vi "Volt Freq Tach Properties.vi"(8 "error in":errorcluster, 10 "MeasType":T1, 11 "Rings Supported In":variant) -> (0 "error out":errorcluster, 3 "Rings Supported Out":variant)   [LabVIEW 2012]
uses:
  Custom Ctrls/ge_MeasType.ctl
  Custom Ctrls/ge_RingSupport.ctl
  Controls/HeaderNames.ctl
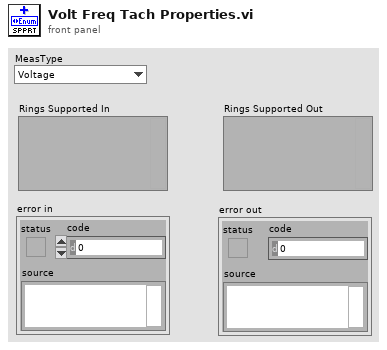
[diagram p1: front panel]
types:
  T1 = typedef "ge_MeasType.ctl" = enum16{"Voltage", "Frequency", "Tachometer", "Dynamic", "Thermocouple", "RTD", "Strain", "Current", "Resistance"}
  T2 = typedef "HeaderNames.ctl" = enum16{"Channel", "Device", "Spacer", "Description", "MB", "Range", "Terminal", "Coupling", "Thresh (V)", "Pulse/Rev", "Slope", "Min EU", "Min RPM", "mV/EU", "Iex", "Temp Units", "Type", "CJC Src", "CJC Val", "Ro", "Wire Cfg", "Strain Mode", "Vex", "Bridge Type", "GF", "Gauge Res", "Poisson", "Lead Res", "Init Strain", "GAF", "Scale", "Offset", "Unit (EU)", "dB?", "dB Ref", "Cal Mag", "Cal Units", "Max Temp", "Min Temp", "Max Strain", "Min Strain"}
  T3 = typedef "ge_RingSupport.ctl" = cluster{"Hdr Name":T2, "Values":u16[]}
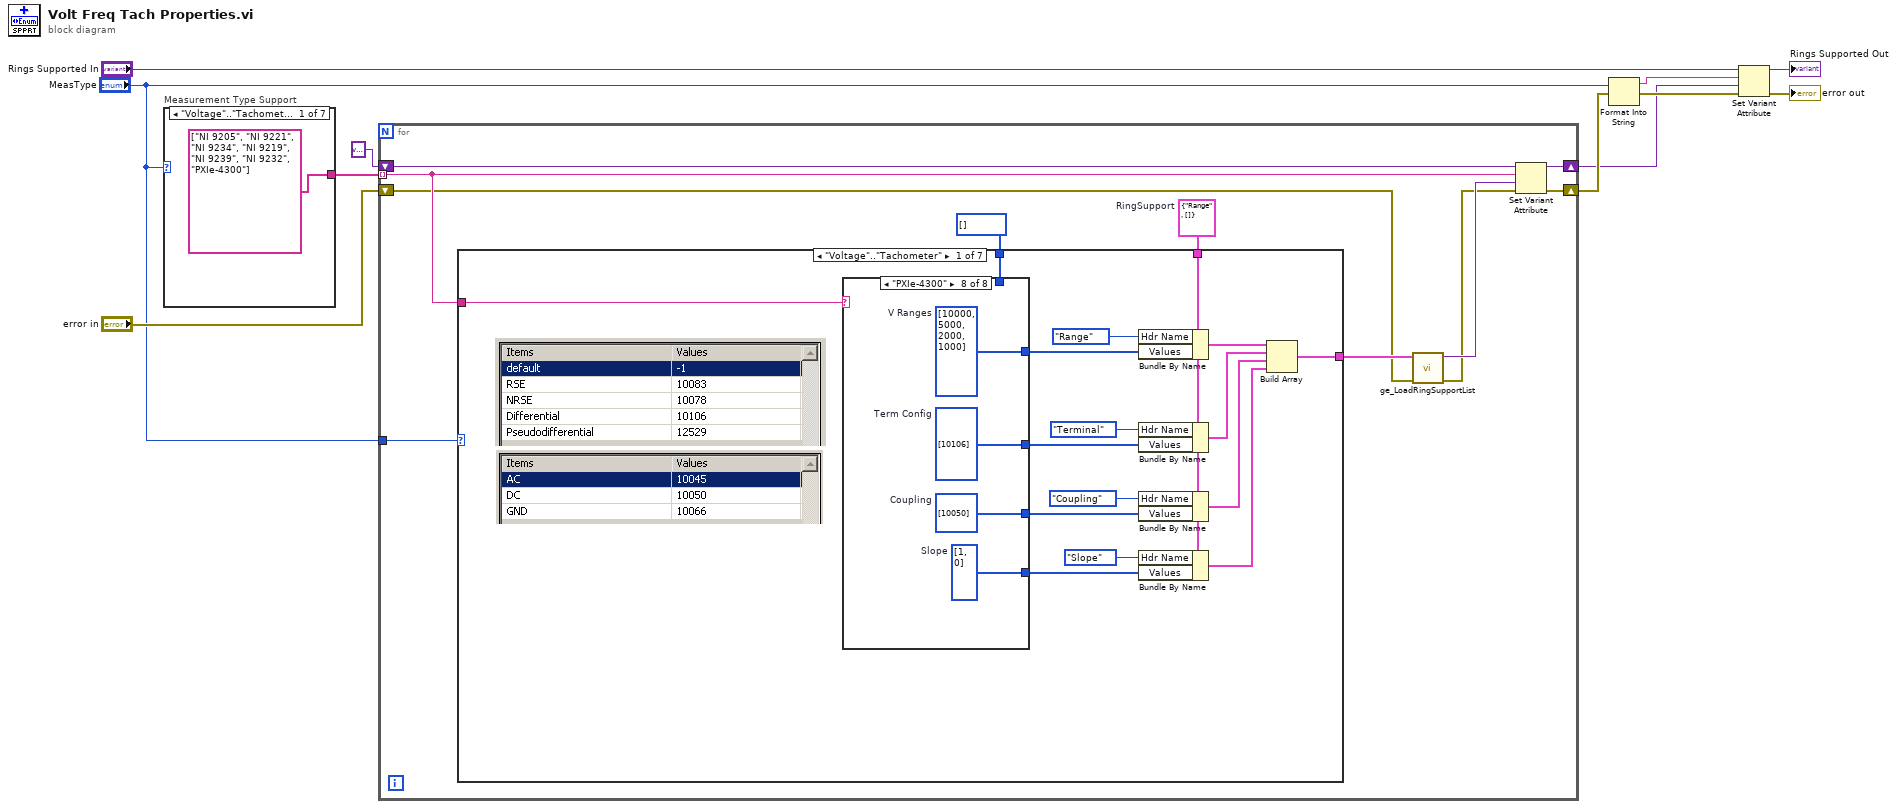
[diagram p0: block diagram]
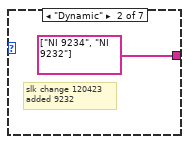
[diagram p2: hidden frame]
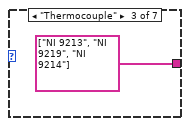
[diagram p3: hidden frame]
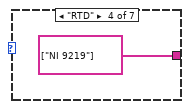
[diagram p4: hidden frame]
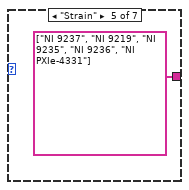
[diagram p5: hidden frame]
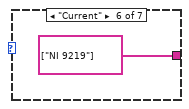
[diagram p6: hidden frame]
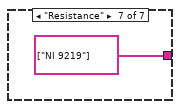
[diagram p7: hidden frame]
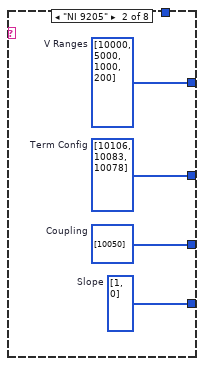
[diagram p9: hidden frame]
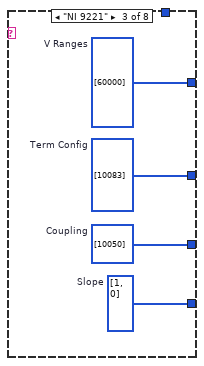
[diagram p10: hidden frame]
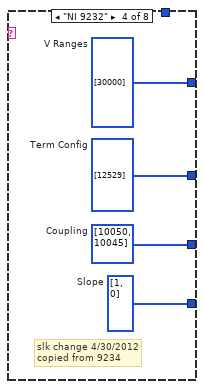
[diagram p11: hidden frame]
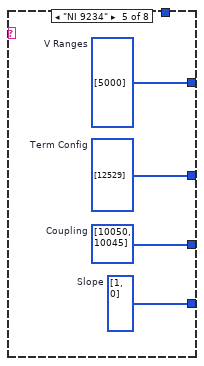
[diagram p12: hidden frame]
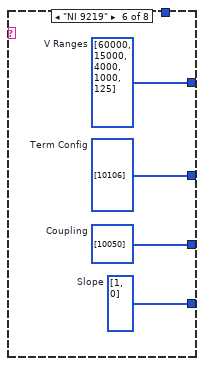
[diagram p13: hidden frame]
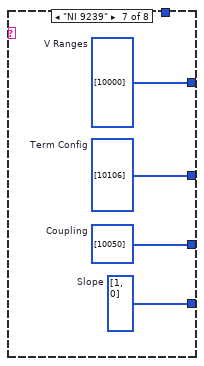
[diagram p14: hidden frame]
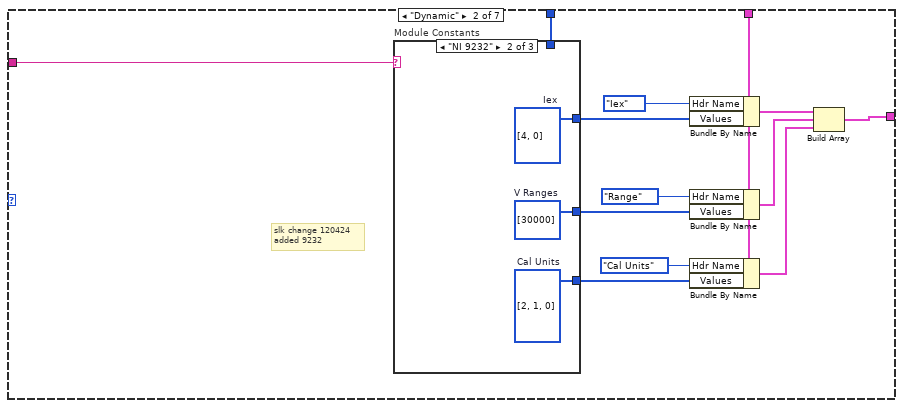
[diagram p15: hidden frame]
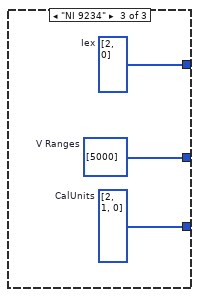
[diagram p17: hidden frame]
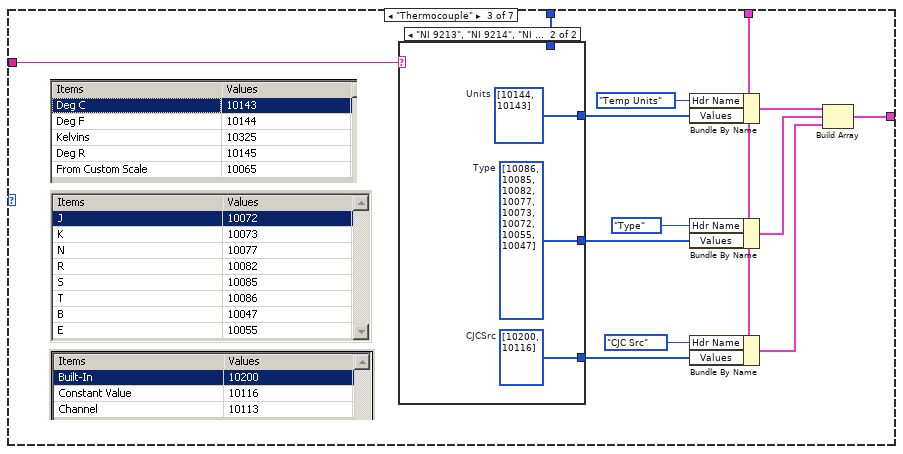
[diagram p18: hidden frame]
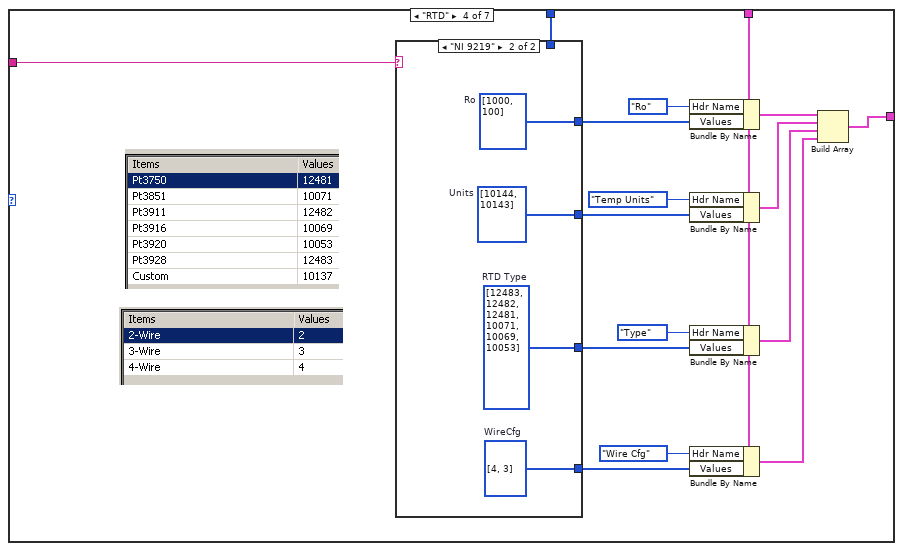
[diagram p20: hidden frame]
diagram:
  n1 = case "Measurement Type Support" shown="\"Voltage\"..\"Tachometer\"" "MeasType" {
    tunnel: [string[] ["NI 9205", "NI 9221", "NI 9234", "NI 9219", "NI 9239", "NI 9232", "PXIe-4300"] string[] ["NI 9234", "NI 9232"] string[] ["NI 9213", "NI 9219", "NI 9214"] string[] ["NI 9219"] string[] ["NI 9237", "NI 9219", "NI 9235", "NI 9236", "NI PXIe-4331"] string[] ["NI 9219"] string[] ["NI 9219"]] -> w11
    frame "Voltage".."Tachometer" {
    }
    frame "Dynamic" {
      # "slk change 120423\nadded 9232"
    }
    frame "Thermocouple" {
    }
    frame "RTD" {
    }
    frame "Strain" {
    }
    frame "Current" {
    }
    frame "Resistance" {
    }
  }
  n2 = for {
    tunnel: w11 -> [w28] mode=indexing
    shift-right: [w24] -> w8
    shift-left: "error in" -> [w23]
    shift-right: [w22] -> w5
    shift-left: variant ("variant") -> [w25]
    tunnel: "MeasType" -> [w19]
    w21 = T3 {"Hdr Name"=enum."Range", "Values"=[]}  # RingSupport
    n3 = case shown="\"Voltage\"..\"Tachometer\"" w19 {
      tunnel: [w33 w77 w98 w114 w135 w162 w170] -> w29
      tunnel: w28 -> [w32 w75 w96 w113 w134 w160 w169]
      tunnel: w21 -> [w31 w78 w97 w115 w136 w161 w171]
      tunnel: u16[] [] ("V Ranges") -> [w30 w76 w95 w112 w133 w159 w168]
      frame "Voltage".."Tachometer" {
        n4 = case shown="\"PXIe-4300\"" w32 {
          tunnel: [w46 w50 w54 w58 w62 w66 w70 w74] -> w41
          tunnel: [w46 w49 w53 w57 w61 w65 w69 w73] -> w40
          tunnel: [w46 w48 w52 w56 w60 w64 w68 w72] -> w39
          tunnel: [w46 w47 w51 w55 w59 w63 w67 w71] -> w38
          tunnel: w30 -> [w46 _ _ _ _ _ _ _]
          frame Default {
          }
          frame "NI 9205" {
            w47 = u16[] [1, 0]  # Slope
            w48 = u16[] [10050]  # Coupling
            w49 = u16[] [10106, 10083, 10078]  # Term Config
            w50 = u16[] [10000, 5000, 1000, 200]  # V Ranges
          }
          frame "NI 9221" {
            w51 = u16[] [1, 0]  # Slope
            w52 = u16[] [10050]  # Coupling
            w53 = u16[] [10083]  # Term Config
            w54 = u16[] [60000]  # V Ranges
          }
          frame "NI 9232" {
            w55 = u16[] [1, 0]  # Slope
            w56 = u16[] [10050, 10045]  # Coupling
            w57 = u16[] [12529]  # Term Config
            w58 = u16[] [30000]  # V Ranges
            # "slk change 4/30/2012\ncopied from 9234"
          }
          frame "NI 9234" {
            w59 = u16[] [1, 0]  # Slope
            w60 = u16[] [10050, 10045]  # Coupling
            w61 = u16[] [12529]  # Term Config
            w62 = u16[] [5000]  # V Ranges
          }
          frame "NI 9219" {
            w63 = u16[] [1, 0]  # Slope
            w64 = u16[] [10050]  # Coupling
            w65 = u16[] [10106]  # Term Config
            w66 = u16[] [60000, 15000, 4000, 1000, 125]  # V Ranges
          }
          frame "NI 9239" {
            w67 = u16[] [1, 0]  # Slope
            w68 = u16[] [10050]  # Coupling
            w69 = u16[] [10106]  # Term Config
            w70 = u16[] [10000]  # V Ranges
          }
          frame "PXIe-4300" {
            w71 = u16[] [1, 0]  # Slope
            w72 = u16[] [10050]  # Coupling
            w73 = u16[] [10106]  # Term Config
            w74 = u16[] [10000, 5000, 2000, 1000]  # V Ranges
          }
        }
        n5 = Bundle By Name(cluster=w31, "Hdr Name"=HeaderNames."Range", "Values"=w41) -> (w37:T3)
        n6 = Bundle By Name(cluster=w31, "Hdr Name"=HeaderNames."Terminal", "Values"=w40) -> (w36:T3)
        n7 = Bundle By Name(cluster=w31, "Hdr Name"=HeaderNames."Coupling", "Values"=w39) -> (w35:T3)
        n8 = Bundle By Name(cluster=w31, "Hdr Name"=HeaderNames."Slope", "Values"=w38) -> (w34:T3)
        n9 = Build Array(w37, w36, w35, w34) -> (w33:T3[])
      }
      frame "Dynamic" {
        # "slk change 120424\nadded 9232"
        n10 = case "Module Constants" shown="\"NI 9232\"" w75 {
          tunnel: [w88 w91 w94] -> w82
          tunnel: [w88 w90 w93] -> w83
          tunnel: [w88 w89 w92] -> w84
          tunnel: w76 -> [w88 _ _]
          frame Default {
          }
          frame "NI 9232" {
            w89 = u16[] [2, 1, 0]  # Cal Units
            w90 = u16[] [30000]  # V Ranges
            w91 = u16[] [4, 0]  # Iex
          }
          frame "NI 9234" {
            w92 = u16[] [2, 1, 0]  # CalUnits
            w93 = u16[] [5000]  # V Ranges
            w94 = u16[] [2, 0]  # Iex
          }
        }
        n11 = Bundle By Name(cluster=w78, "Hdr Name"=HeaderNames."Iex", "Values"=w82) -> (w85:T3)
        n12 = Bundle By Name(cluster=w78, "Hdr Name"=HeaderNames."Range", "Values"=w83) -> (w86:T3)
        n13 = Bundle By Name(cluster=w78, "Hdr Name"=HeaderNames."Cal Units", "Values"=w84) -> (w87:T3)
        n14 = Build Array(w85, w86, w87) -> (w77:T3[])
      }
      frame "Thermocouple" {
        n15 = case shown="\"NI 9213\", \"NI 9214\", \"NI 9219\"" w96 {
          tunnel: [w108 w110] -> w102
          tunnel: [w108 w111] -> w103
          tunnel: [w108 w109] -> w104
          tunnel: w95 -> [w108 _]
          frame Default {
          }
          frame "NI 9213", "NI 9214", "NI 9219" {
            w109 = u16[] [10200, 10116]  # CJCSrc
            w111 = u16[] [10086, 10085, 10082, 10077, 10073, 10072, 10055, 10047]  # Type
            w110 = u16[] [10144, 10143]  # Units
          }
        }
        n16 = Bundle By Name(cluster=w97, "Hdr Name"=HeaderNames."Temp Units", "Values"=w102) -> (w105:T3)
        n17 = Bundle By Name(cluster=w97, "Hdr Name"=HeaderNames."Type", "Values"=w103) -> (w106:T3)
        n18 = Bundle By Name(cluster=w97, "Hdr Name"=HeaderNames."CJC Src", "Values"=w104) -> (w107:T3)
        n19 = Build Array(w105, w106, w107) -> (w98:T3[])
      }
      frame "RTD" {
        n20 = case shown="\"NI 9219\"" w113 {
          tunnel: [w128 w129] -> w120
          tunnel: [w128 w130] -> w121
          tunnel: [w128 w131] -> w122
          tunnel: [w128 w132] -> w123
          tunnel: w112 -> [w128 _]
          frame Default {
          }
          frame "NI 9219" {
            w132 = u16[] [4, 3]  # WireCfg
            w131 = u16[] [12483, 12482, 12481, 10071, 10069, 10053]  # RTD Type
            w130 = u16[] [10144, 10143]  # Units
            w129 = u16[] [1000, 100]  # Ro
          }
        }
        n21 = Bundle By Name(cluster=w115, "Hdr Name"=HeaderNames."Ro", "Values"=w120) -> (w124:T3)
        n22 = Bundle By Name(cluster=w115, "Hdr Name"=HeaderNames."Temp Units", "Values"=w121) -> (w125:T3)
        n23 = Bundle By Name(cluster=w115, "Hdr Name"=HeaderNames."Type", "Values"=w122) -> (w126:T3)
        n24 = Bundle By Name(cluster=w115, "Hdr Name"=HeaderNames."Wire Cfg", "Values"=w123) -> (w127:T3)
        n25 = Build Array(w124, w125, w126, w127) -> (w114:T3[])
      }
      frame "Strain" {
        # "Mode:\nHigh Res 0 \nHigh Range 1"
        n26 = case shown="\"NI 9236\"" w134 {
          tunnel: [w146 w147 w152 w155 w158] -> w140
          tunnel: [w146 w149 w151 w154 w157] -> w141
          tunnel: [w146 w148 w150 w153 w156] -> w142
          tunnel: w133 -> [w146 _ _ _ _]
          frame Default {
          }
          frame "NI 9237" {
            w147 = u16[] [0]  # Mode
            w148 = u16[] [10272, 10271, 10189, 10188, 10185, 10184, 10183]  # Type
            w149 = u16[] [10000, 5000, 3300, 2500]  # Vex
          }
          frame "NI 9219" {
            w150 = u16[] [10272, 10271, 10189, 10188, 10185, 10184, 10183]  # Type
            w151 = u16[] [2500]  # Vex
            w152 = u16[] [1, 0]  # Mode
          }
          frame "NI 9235" {
            w153 = u16[] [10271]  # Type
            w154 = u16[] [2000]  # Vex
            w155 = u16[] [1]  # Mode
          }
          frame "NI 9236" {
            w156 = u16[] [10271]  # Type
            w157 = u16[] [3300]  # Vex
            w158 = u16[] [1]  # Mode
          }
        }
        n27 = Bundle By Name(cluster=w136, "Hdr Name"=HeaderNames."Strain Mode", "Values"=w140) -> (w143:T3)
        n28 = Bundle By Name(cluster=w136, "Hdr Name"=HeaderNames."Vex", "Values"=w141) -> (w144:T3)
        n29 = Bundle By Name(cluster=w136, "Hdr Name"=HeaderNames."Bridge Type", "Values"=w142) -> (w145:T3)
        n30 = Build Array(w143, w144, w145) -> (w135:T3[])
      }
      frame "Current" {
        n31 = case shown="\"NI 9219\"" w160 {
          tunnel: [w166 w167] -> w164
          tunnel: w159 -> [w166 _]
          frame Default {
          }
          frame "NI 9219" {
            w167 = u16[] [25]  # Ro
          }
        }
        n32 = Bundle By Name(cluster=w161, "Hdr Name"=HeaderNames."Range", "Values"=w164) -> (w165:T3)
        n33 = Build Array(w165) -> (w162:T3[])
      }
      frame "Resistance" {
        n34 = case shown="\"NI 9219\"" w169 {
          tunnel: [w178 w180] -> w174
          tunnel: [w178 w179] -> w175
          tunnel: w168 -> [w178 _]
          frame Default {
          }
          frame "NI 9219" {
            w179 = u16[] [4, 2]  # Wire Config
            w180 = u16[] [10000, 1000]  # O Range
          }
        }
        n35 = Bundle By Name(cluster=w171, "Hdr Name"=HeaderNames."Range", "Values"=w174) -> (w176:T3)
        n36 = Bundle By Name(cluster=w171, "Hdr Name"=HeaderNames."Wire Cfg", "Values"=w175) -> (w177:T3)
        n37 = Build Array(w176, w177) -> (w170:T3[])
      }
    }
    n38 = call "ge_LoadRingSupportList.vi"("error in"=w23, "RingSupport"=w29) -> ("error out"=w26:errorcluster, "List Variant"=w27:variant)  [unwired: 8 in]
    n39 = Set Variant Attribute(Variant=w25, name=w28, value=w27, error in=w26) -> (Variant out=w22:variant, error out=w24:errorcluster)  [unwired: 1 out]
  }
  n40 = Format Into String(error in=w8, "MeasType") -> (resulting string=w6:string, error out=w7:errorcluster)  [unwired: 2 in]
  n41 = Set Variant Attribute(Variant="Rings Supported In", name=w6, value=w5, error in=w7) -> (Variant out=→"Rings Supported Out":variant, error out=→"error out":errorcluster)  [unwired: 1 out]
